vi "SSL Detection Robot.vi"(8 "error in":errorcluster, 9 "Array":u8[](array[numeric]) format="%02x") -> (0 "error out":errorcluster, 1 "Length-delimited":u8[](array[numeric]) format="%02x", 3 "Detection Robot":T1)   [LabVIEW 2016]
uses:
  SSL Detection Robot.ctl
  Varint Decoder uint32.vi
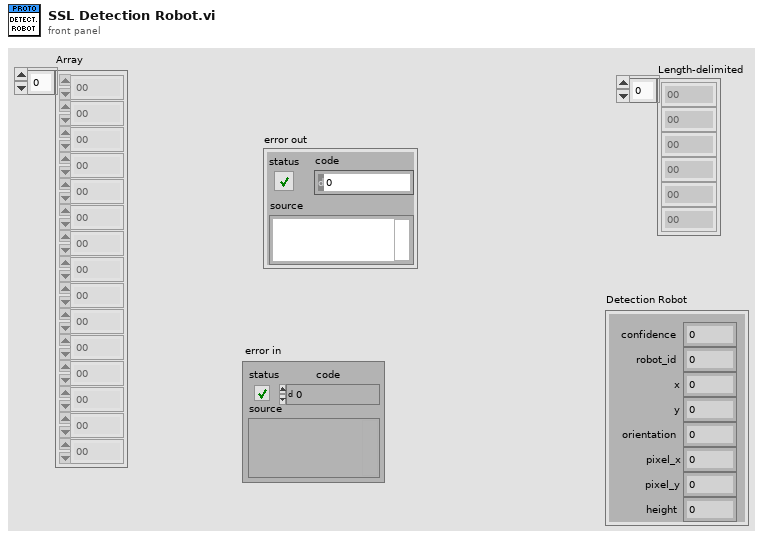
[diagram p1: front panel]
types:
  T1 = typedef "SSL Detection Robot.ctl" = cluster{"x":dbl, "robot_id":u32, "confidence":sgl, "y":sgl, "orientation":sgl, "pixel_x":sgl, "pixel_y":sgl, "height":sgl}
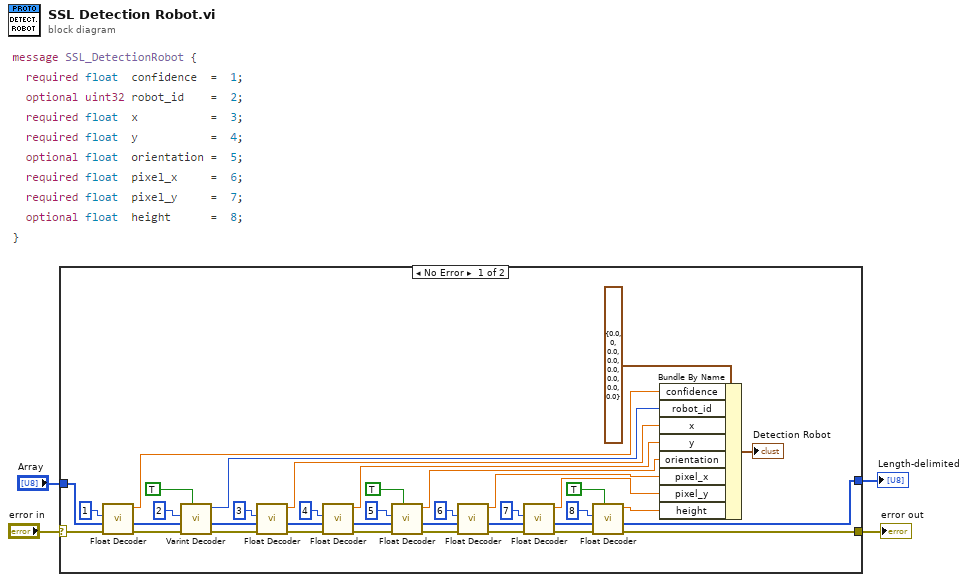
[diagram p0: block diagram]
diagram:
  n1 = case shown="No Error" "error in" {
    selector: "error in" -> [w42 w45]
    tunnel: [w18 w45] -> w3
    tunnel: [w19 w44] -> w2
    tunnel: "Array" -> [w6 w44]
    frame No Error {
      n2 = call "Float Decoder.vi"("error in (no error)"=w42, "Array"=w6, "Key"=1) -> ("error out"=w41:errorcluster, "array w/ subset deleted"=w5:u8[], "Float"=w29:sgl)  [unwired: 5 in, 1 out]
      n3 = call-poly "Varint Decoder.vi"("Optional"=TRUE, "error in (no error)"=w41, "Array"=w5, "Key"=2) -> ("error out"=w40:errorcluster, "array w/ subset deleted"=w8:u8[], "Varint"=w28:u32)  [unwired: 4 in, 1 out]
      n4 = call "Float Decoder.vi"("error in (no error)"=w40, "Array"=w8, "Key"=3) -> ("error out"=w39:errorcluster, "array w/ subset deleted"=w9:u8[], "Float"=w27:sgl)  [unwired: 5 in, 1 out]
      n5 = call "Float Decoder.vi"("error in (no error)"=w39, "Array"=w9, "Key"=4) -> ("error out"=w34:errorcluster, "array w/ subset deleted"=w10:u8[], "Float"=w26:sgl)  [unwired: 5 in, 1 out]
      n6 = call "Float Decoder.vi"("Optional"=TRUE, "error in (no error)"=w34, "Array"=w10, "Key"=5) -> ("error out"=w32:errorcluster, "array w/ subset deleted"=w12:u8[], "Float"=w25:sgl)  [unwired: 4 in, 1 out]
      n7 = call "Float Decoder.vi"("error in (no error)"=w32, "Array"=w12, "Key"=6) -> ("error out"=w30:errorcluster, "array w/ subset deleted"=w13:u8[], "Float"=w24:sgl)  [unwired: 5 in, 1 out]
      n8 = call "Float Decoder.vi"("error in (no error)"=w30, "Array"=w13, "Key"=7) -> ("error out"=w21:errorcluster, "array w/ subset deleted"=w14:u8[], "Float"=w23:sgl)  [unwired: 5 in, 1 out]
      n9 = call "Float Decoder.vi"("Optional"=TRUE, "error in (no error)"=w21, "Array"=w14, "Key"=8) -> ("error out"=w18:errorcluster, "array w/ subset deleted"=w19:u8[], "Float"=w20:sgl)  [unwired: 4 in, 1 out]
      n10 = Bundle By Name(cluster=T1 {"x"=0.0, "robot_id"=0, "confidence"=0.0, "y"=0.0, "orientation"=0.0, "pixel_x"=0.0, "pixel_y"=0.0, "height"=0.0} ("Detection Robot 2"), "confidence"=w29, "robot_id"=w28, "x"=w27, "y"=w26, "orientation"=w25, "pixel_x"=w24, "pixel_y"=w23, "height"=w20) -> (→"Detection Robot":T1)
    }
    frame Error {
    }
  }
  "error out" <- w3
  "Length-delimited" <- w2
